vi "Set Export Setup (Temp).vi"(8 "error in (no error)":errorcluster, 9 "Export Setup":T2[](array[typedef]), 11 "Map":T1) -> (0 "error out":errorcluster, 3 "Map Out":T1)   [LabVIEW 2015, in "ConfigHelper.lvlib"]
uses:
  ConfigHelper.lvlib
  Control_Export Setup.ctl
  <vilib>/addons/PointValueMap/controls/PointMap.ctl
  <vilib>/addons/PointValueMap/subVIs/Point_Write_variant.vi
  <vilib>/addons/PointValueMap/PointValueMap.lvlib
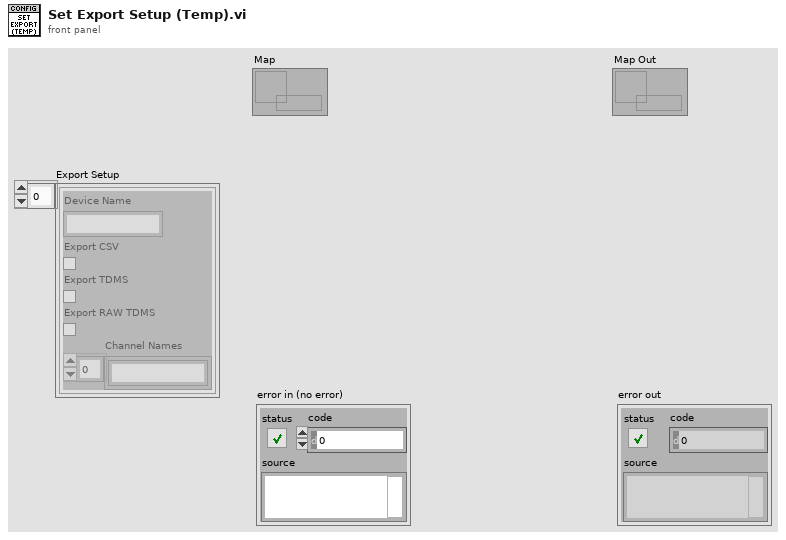
[diagram p1: front panel]
types:
  T1 = typedef "PointValueMap.lvlib/PointMap.ctl" = refnum<data-value>
  T2 = typedef "ConfigHelper.lvlib/Control_Export Setup.ctl" = cluster{"Device Name":string, "Export CSV":bool, "Export TDMS":bool, "Export RAW TDMS":bool, "Channel Names":string[]}
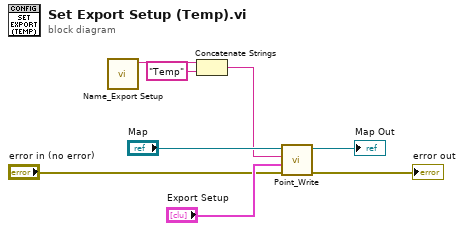
[diagram p0: block diagram]
diagram:
  n1 = call "Name_Export Setup.vi"() -> ("Name"=w3:string)  [unwired: 11 in]
  n2 = Concatenate Strings(w3, "Temp" ("string")) -> (w1:string)
  n3 = call-poly <vilib>:"Point_Write.vi"("Error In"="error in (no error)", "Value"="Export Setup", "Tag"=w1, "Map"="Map") -> ("Error Out"=→"error out":errorcluster, "Map Out"=→"Map Out":T1)  [unwired: 6 in]
